vi "Notify.vi"(8 "error in (no error)":errorcluster, 10 "ErrorOrSuccess":refnum<class "ErrorOrSuccess.lvclass">, 11 "Unsubscribe JSON in":refnum<class "Unsubscribe JSON.lvclass">) -> (0 "error out":errorcluster, 3 "Unsubscribe JSON out":refnum<class "Unsubscribe JSON.lvclass">)   [LabVIEW 2020, in "wamplv.lvlib" / "Unsubscribe JSON.lvclass"]
uses:
  Unsubscribe JSON.lvclass
  Unsubscribe JSON.lvclass/Unsubscribe JSON.ctl
  WAMP Client/API/TypeDefs/Error or abort detail (JSON).ctl
  wamplv.lvlib
  WAMP Client/Private/TypeDef/UNSUBSCRIBE Result (JSON).ctl
  Message loop classes/ErrorOrSuccess/ErrorOrSuccess.lvclass
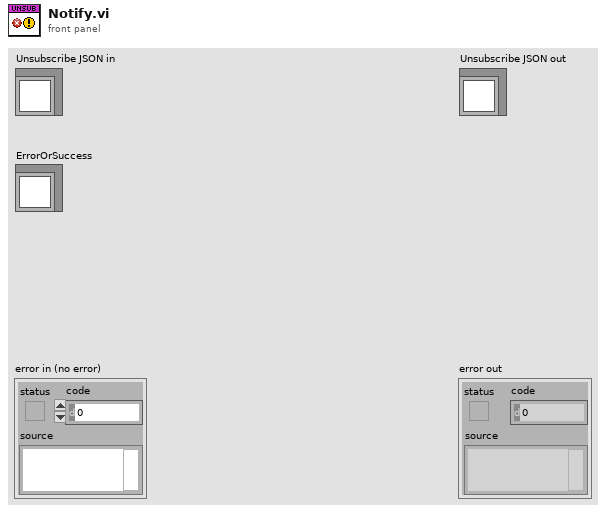
[diagram p1: front panel]
types:
  T1 = typedef "wamplv.lvlib/UNSUBSCRIBE Result (JSON).ctl" = cluster{"Success?":bool, "Error/Abort details (JSON)":T2}
  T2 = typedef "wamplv.lvlib/Error or abort detail (JSON).ctl" = cluster{"Error URI":string, "Error Arguments":string, "Error ArgumentKw":string, "Error Details":string, "Associated LabVIEW Error":errorcluster}
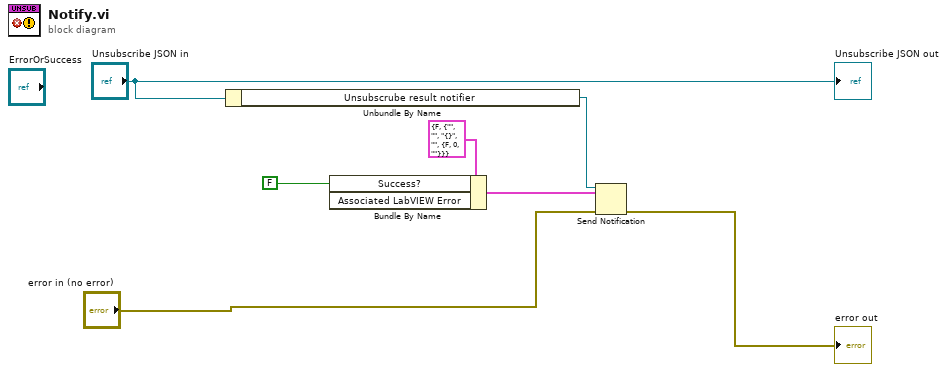
[diagram p0: block diagram]
diagram:
  n1 = Unbundle By Name("Unsubscribe JSON in") -> ("Unsubscrube result notifier"=w1:refnum<notifier>)
  n2 = Bundle By Name(cluster=T1 {"Success?"=FALSE, "Error/Abort details (JSON)"={"Error URI"="", "Error Arguments"="", "Error ArgumentKw"="{}", "Error Details"="", "Associated LabVIEW Error"={"status"=FALSE, "code"=0, "source"=""}}} ("Unsubcsribe Result"), "Success?"=FALSE) -> (w3:T1, "Associated LabVIEW Error"=w6:errorcluster)
  n3 = Send Notification(notification=w3, notifier=w1, error in (no error)="error in (no error)") -> (error out=→"error out":errorcluster)  [unwired: 1 out]
  "Unsubscribe JSON out" <- "Unsubscribe JSON in"
